vi "OPERACIONES.vi"() -> ()   [LabVIEW 2016]
panel:
  in  "stop":bool
  out "DIVISION":dbl
  out "MULTIPLICACION":dbl
  out "RESTA":dbl
  out "SUMA":dbl
  in  "NUMERO 2":dbl
  in  "NUMERO 1":dbl
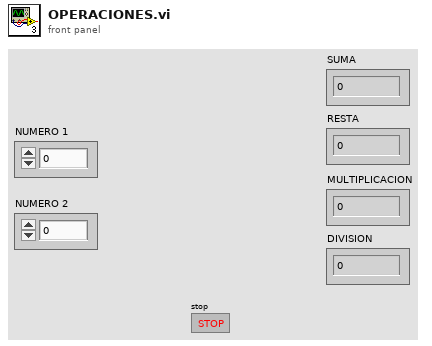
[diagram p1: front panel]
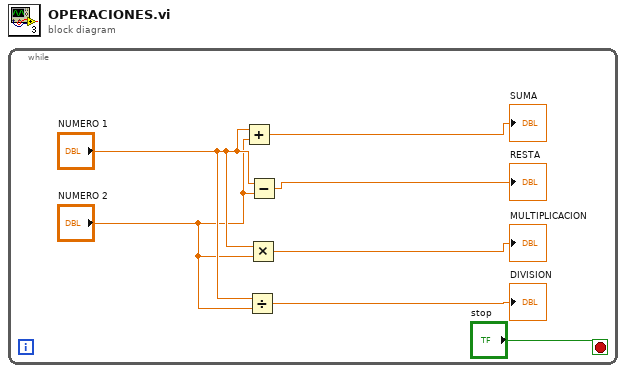
[diagram p0: block diagram]
diagram:
  n1 = while {
    stop <- "stop" stop-if-true
    n2 = Add(x="NUMERO 1", y="NUMERO 2") -> (x+y=→"SUMA":dbl)
    n3 = Divide(x="NUMERO 1", y="NUMERO 2") -> (x/y=→"DIVISION":dbl)
    n4 = Multiply(x="NUMERO 1", y="NUMERO 2") -> (x*y=→"MULTIPLICACION":dbl)
    n5 = Subtract(x="NUMERO 1", y="NUMERO 2") -> (x-y=→"RESTA":dbl)
  }
